vi "genSenA.vi"(8 "error in (no error)":errorcluster, 10 "Field Idx":i32[](array[numeric]), 11 "OptStateEsti in":refnum<class "OptStateEsti.lvclass">) -> (0 "error out":errorcluster, 2 "Stacked 2D Array":dbl[][](array[numeric]), 3 "OptStateEsti out":refnum<class "OptStateEsti.lvclass">)   [LabVIEW 2016, in "OptStateEsti.lvclass"]
doc: "Generate the sensitivity matrix A based on the array of field index."
uses:
  OptStateEsti.lvclass
  OptStateEsti.lvclass/OptStateEsti.ctl
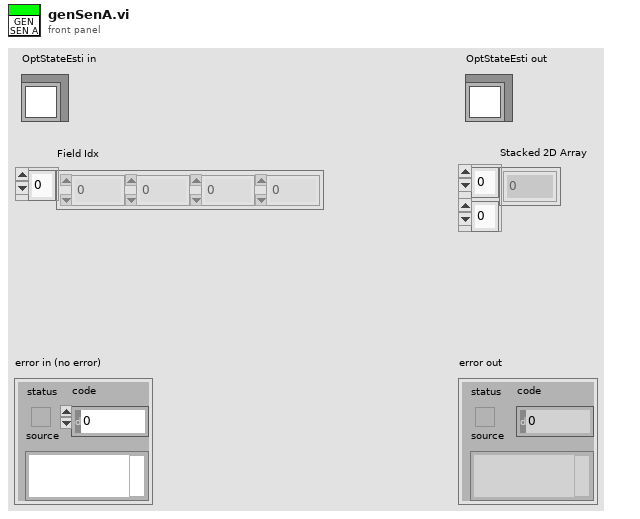
[diagram p1: front panel]
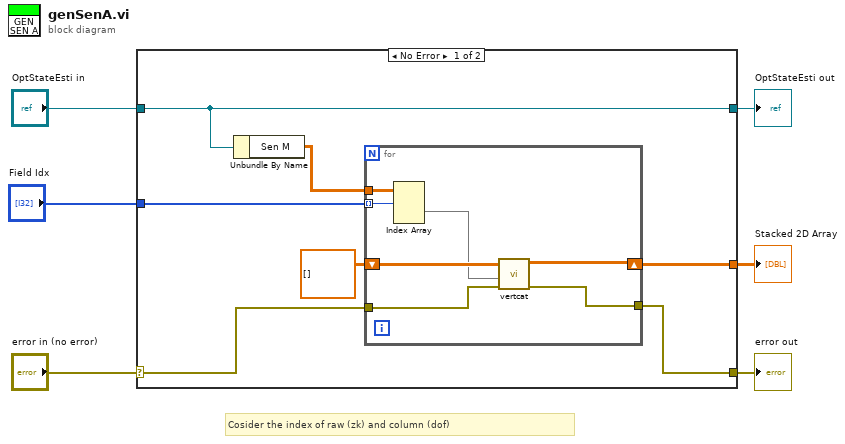
[diagram p0: block diagram]
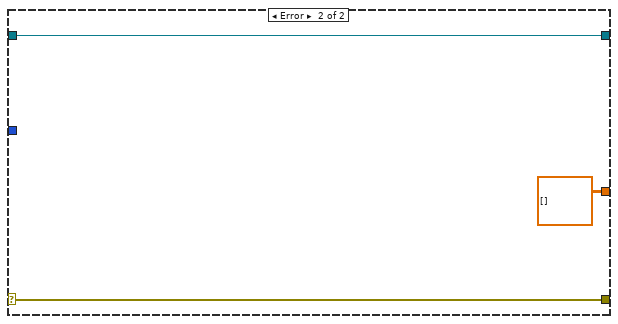
[diagram p2: hidden frame]
diagram:
  # "Cosider the index of raw (zk) and column (dof)"
  n1 = case shown="No Error" "error in (no error)" {
    selector: "error in (no error)" -> [w8 w23]
    tunnel: [w7 w23] -> w5
    tunnel: [w13 w22] -> w3
    tunnel: "OptStateEsti in" -> [w13 w22]
    tunnel: "Field Idx" -> [w11 _]
    tunnel: [w9 dbl[][] [] ("Stacked 2D Array")] -> w1
    frame No Error {
      n2 = Unbundle By Name(w13) -> ("Sen M"=w12:dbl[][][])
      n3 = for {
        tunnel: w12 -> [w20]
        tunnel: w11 -> [w19] mode=indexing
        shift-right: [w17] -> w9
        shift-left: dbl[][] [] ("Stacked 2D Array") -> [w18]
        tunnel: w8 -> [w15]
        tunnel: [w14] -> w7
        n4 = Index Array(array=w20, index (dim 0)=w19) -> (element=w16:dbl[][])  [unwired: 2 in]
        n5 = call "vertcat.vi"("error in (no error)"=w15, "A1"=w16, "A0"=w18) -> ("error out"=w14:errorcluster, "Stacked 2D Array"=w17:dbl[][])  [unwired: 7 in]
      }
    }
    frame Error {
    }
  }
  "error out" <- w5
  "OptStateEsti out" <- w3
  "Stacked 2D Array" <- w1
